vi "2-input X-NOR.vi"(10 "Obtained Expression":string, 11 "Input List":string[](array[string])) -> (2 "X-NOR ?":bool, 3 "Logic Exp":string)   [LabVIEW 2014]
doc: "This VI is used to compare the obtained logic with the logic of NAND gate."
panel:
  out "concatenated string":string
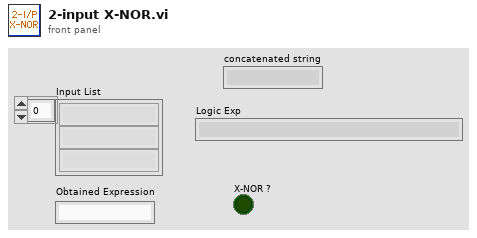
[diagram p1: front panel]
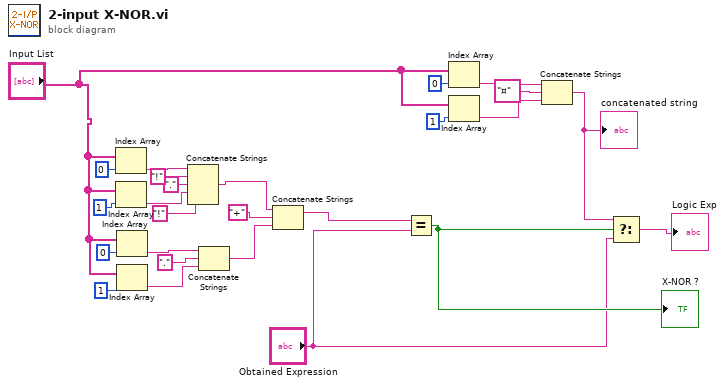
[diagram p0: block diagram]
diagram:
  n1 = Index Array(array="Input List", index=0) -> (element=w17:string)
  n2 = Index Array(array="Input List", index=1) -> (element=w14:string)
  n3 = Index Array(array="Input List", index=0) -> (element=w23:string)
  n4 = Index Array(array="Input List", index=1) -> (element=w25:string)
  n5 = Concatenate Strings(w17, "!" ("t"), "." ("string"), w14, "!" ("t")) -> (w19:string)
  n6 = Concatenate Strings(w23, "." ("string"), w25) -> (w26:string)
  n7 = Concatenate Strings(w19, "+" ("string"), w26) -> (w13:string)
  n8 = Equal?(x=w13, y="Obtained Expression") -> (x = y?=w12:bool)
  "X-NOR ?" <- w12
  n9 = Index Array(array="Input List", index=0) -> (element=w8:string)
  n10 = Index Array(array="Input List", index=1) -> (element=w6:string)
  n11 = Concatenate Strings(w8, "¤" ("string"), w6) -> (w5:string)
  "concatenated string" <- w5
  n12 = Select(t=w5, s=w12, f="Obtained Expression") -> (s? t:f=→"Logic Exp":string)
